vi "Write D-Register.vi"(8 "error in":errorcluster, 9 "Data":u32, 10 "D-register number":u32=1, 11 "VISA resource name":refnum<visa-resource-name>) -> (0 "error out":errorcluster, 2 "Successfully":bool, 3 "VISA resource name out":refnum<visa-resource-name>)   [LabVIEW 2017, in "Samwontech TEMP2xxx.lvlib"]
doc: "WSD command is used to write data to a part of D-Register by consecutive address in sequence."
uses:
  <instrlib>/Samwontech TEMP2xxx/Samwontech TEMP2xxx.lvlib
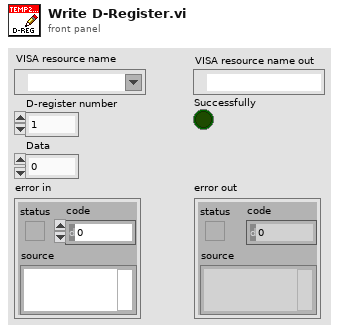
[diagram p1: front panel]
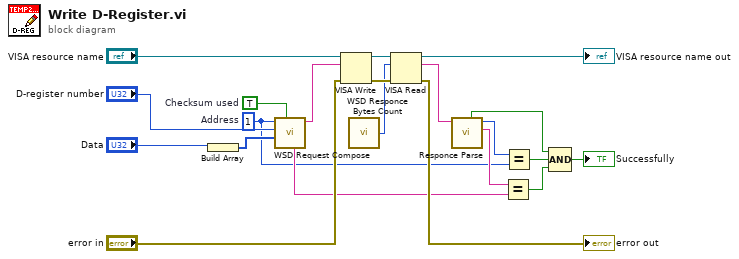
[diagram p0: block diagram]
diagram:
  w5 = u8 1  # Address
  w21 = TRUE  # Checksum used
  n1 = Build Array("Data") -> (w18:u32[])
  n2 = call <instrlib>:"WSD Request Compose.vi"("Checksum used"=w21, "Data"=w18, "D-register number"="D-register number", "Address"=w5) -> ("Request"=w10:string, "Command"=w7:string)  [unwired: 6 in]
  n3 = VISA Write(VISA resource name="VISA resource name", write buffer=w10, error in (no error)="error in") -> (VISA resource name out=w11:refnum<visa-resource-name>, error out=w17:errorcluster)  [unwired: 1 out]
  n4 = call <instrlib>:"WSD Responce Bytes Count.vi"() -> ("Bytes Count"=w12:u32)
  n5 = VISA Read(VISA resource name=w11, byte count=w12, error in (no error)=w17) -> (VISA resource name out=→"VISA resource name out":refnum<visa-resource-name>, read buffer=w9:string, error out=→"error out":errorcluster)  [unwired: 1 out]
  n6 = call <instrlib>:"Responce Parse.vi"("Responce"=w9) -> ("Command"=w8:string, "Address"=w6:u8, "OK"=w2:bool)  [unwired: 6 in, 2 out]
  n7 = Equal?(x=w8, y=w7) -> (x = y?=w4:bool)
  n8 = Equal?(x=w6, y=w5) -> (x = y?=w3:bool)
  n9 = Compound Arithmetic op=AND(w2, w3, w4) -> (→"Successfully":bool)
